vi "Save Image & Message Box Flir-Ax8.vi"(1 "Image":T1) -> ()   [LabVIEW 2016]
uses:
  <vilib>/vision/Image Controls.llb/IMAQ Image.ctl
  Type Def Flir-Ax8.ctl
  Global Flir-Ax8.vi
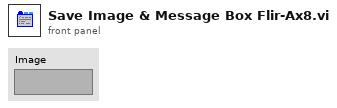
[diagram p1: front panel]
types:
  T1 = typedef "IMAQ Image.ctl" = refnum<image>
  T2 = typedef "Type Def Flir-Ax8.ctl" = enum16{"Initialize", "Save image", "Message box", "Exit"}
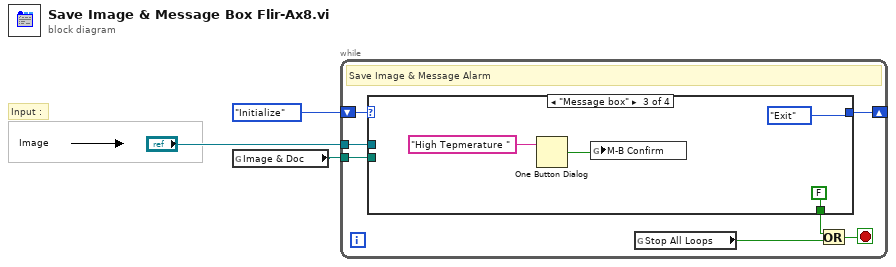
[diagram p0: block diagram]
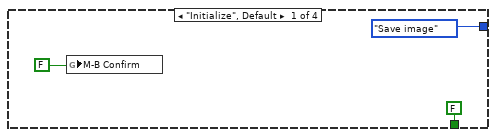
[diagram p2: hidden frame]
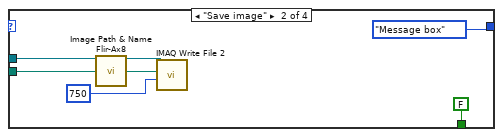
[diagram p3: hidden frame]
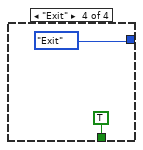
[diagram p4: hidden frame]
diagram:
  # "Input :"
  n1 = global read "Global Flir-Ax8.vi" "Image & Doc"() -> (w1:path)
  n2 = while {
    shift-right: [w8] -> _
    shift-left: Type_Def_Flir-Ax8."Initialize" -> [w9]
    tunnel: w1 -> [w7]
    tunnel: "Image" -> [w6]
    stop <- w5 stop-if-true
    # "Save Image & Message Alarm"
    n3 = case shown="\"Message box\"" w9 {
      tunnel: [FALSE FALSE FALSE TRUE] -> w10
      tunnel: [Type_Def_Flir-Ax8."Save image" Type_Def_Flir-Ax8."Message box" Type_Def_Flir-Ax8."Exit" Type_Def_Flir-Ax8."Exit"] -> w8
      tunnel: w7 -> [_ w17 _ _]
      tunnel: w6 -> [_ w16 _ _]
      frame "Initialize", Default {
        n4 = global write "Global Flir-Ax8.vi" "M-B Confirm"(FALSE ("M-B User Confirmation.")) -> ()
      }
      frame "Save image" {
        n5 = call "Image Path & Name Flir-Ax8.vi"("Base Path"=w17) -> ("Appended Path"=w18:path)
        n6 = call-poly "IMAQ Write File 2"("Image Quality"=u32 750, "File Path"=w18, "Image"=w16) -> ()  [unwired: 7 in, 2 out]
      }
      frame "Message box" {
        n7 = One Button Dialog(message="High Tepmerature ") -> (true=w21:bool)  [unwired: 1 in]
        n8 = global write "Global Flir-Ax8.vi" "M-B Confirm"(w21) -> ()
      }
      frame "Exit" {
      }
    }
    n9 = global read "Global Flir-Ax8.vi" "Stop All Loops"() -> (w4:bool)
    n10 = Or(x=w10, y=w4) -> (x .or. y?=w5:bool)
  }
